vi "ElevFF_MaxAchieveAccel.vi"(9 "Velocity":dbl, 10 "MaxVoltage":dbl, 11 "in ELEV_FF":T1 {"Kg" format="%13.5p"; "Ka" format="%13.5p"; "Kv" format="%13.5p"; "Ks" format="%13.5p"}) -> (3 "MaxAccel":dbl)   [LabVIEW 2019, in "Trajectory_Library.lvlib"]
doc: "Calculates the maximum achievable acceleration given a maximum voltage supply and a velocity. Useful for ensuring that velocity and acceleration constraints for a trapezoidal profile are simultaneously achievable - enter the velocity constraint, and this will give you a simultaneously-achievable acceleration constraint.\n \nInputs: \n - ElevFF -- The ElevFF data cluster\n - maxVoltage -- The maximum voltage that can be supplied to the elevator.\n - velocity -- The velocity of the elevator.\n\nOutputs:\n - MaxAccel -- The maximum possible acceleration at the given velocity."
uses:
  Trajectory_Library.lvlib
  TypeDef/ELEV_FF.ctl
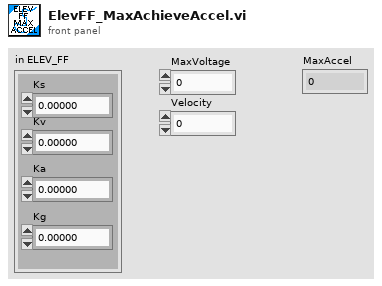
[diagram p1: front panel]
types:
  T1 = typedef "Trajectory_Library.lvlib/ELEV_FF.ctl" = cluster{"Ks":dbl, "Kv":dbl, "Ka":dbl, "Kg":dbl}
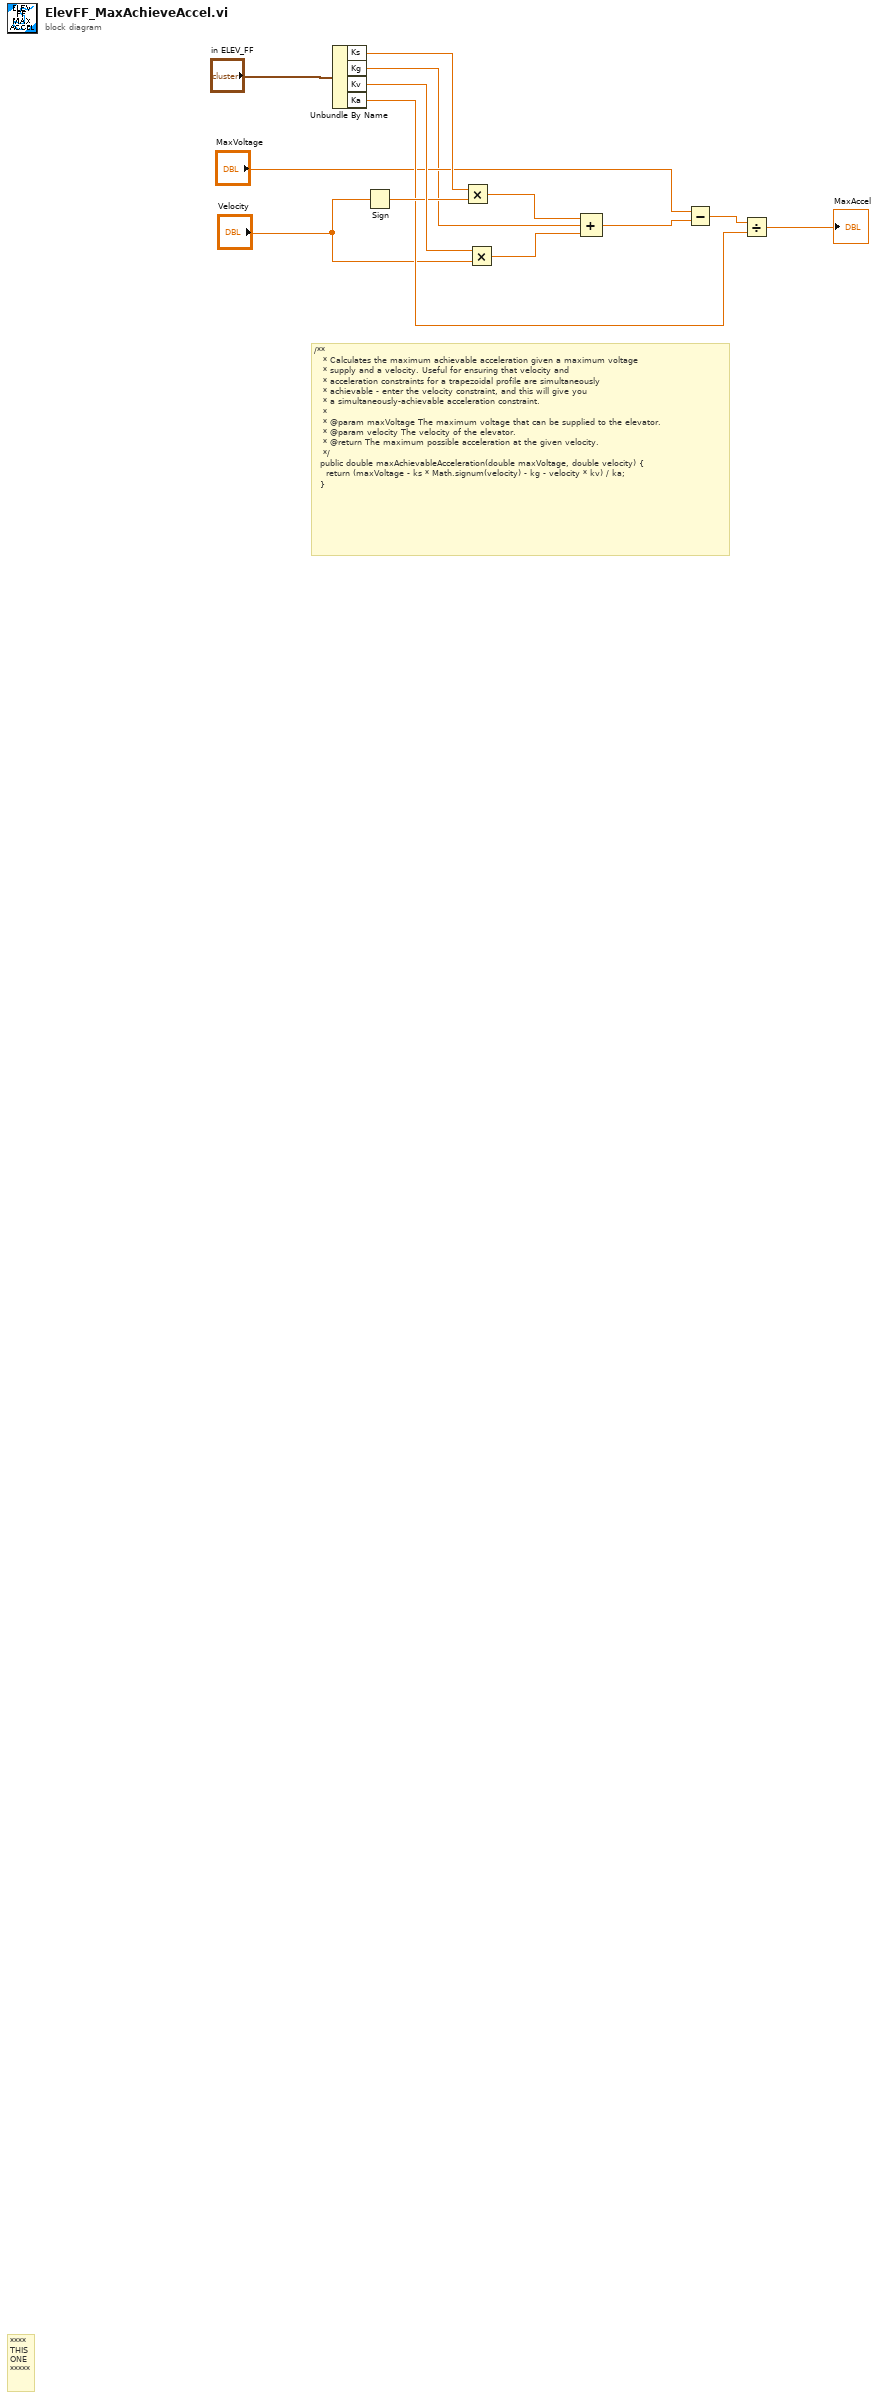
[diagram p0: block diagram]
diagram:
  # "/**\n   * Calculates the maximum achievable acceleration given a maximum voltage\n   * supply and a velocity. Useful for ensuring that velocity and\n   * acceleration constraints for a trapezoidal profile are simultaneously\n   * achievable - enter the velocity constraint, and this will give you\n   * a simultaneously-achievable acceleration constraint.\n   *\n   * @param maxVoltage The maximum voltage that can be supplied to the elevator.\n   * @param velocity The velocity of the elevator.\n   * @return The maximum possible acceleration at the given velocity.\n   */\n  public double maxAchievableAcceleration(double maxVoltage, double velocity) {\n    return (maxVoltage - ks * Math.signum(velocity) - kg - velocity * kv) / ka;\n  }"
  # "****\nTHIS\nONE\n*****"
  n1 = Unbundle By Name("in ELEV_FF") -> ("Ks"=w10:dbl, "Kg"=w2:dbl, "Kv"=w9:dbl, "Ka"=w4:dbl)
  n2 = Sign(1:"Velocity") -> (0:w8:dbl)
  n3 = Multiply(x=w10, y=w8) -> (x*y=w12:dbl)
  n4 = Multiply(x=w9, y="Velocity") -> (x*y=w11:dbl)
  n5 = Compound Arithmetic op=ADD(w12, w2, w11) -> (w7:dbl)
  n6 = Subtract(x="MaxVoltage", y=w7) -> (x-y=w6:dbl)
  n7 = Divide(x=w6, y=w4) -> (x/y=→"MaxAccel":dbl)
